vi "Get Label Text and Index.vi"(0 "Label Text and Index":string) -> (4 "Label Text and Index (Dup)":string, 8 "Text":string, 15 "Index":i32)   [LabVIEW 2016]
uses:
  <vilib>/regexp/Match Regular Expression.xnode
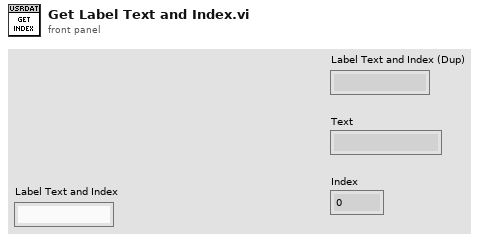
[diagram p1: front panel]
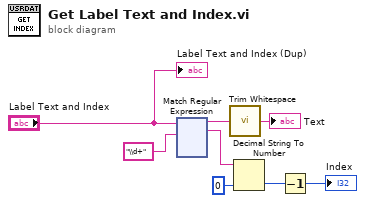
[diagram p0: block diagram]
diagram:
  n1 = xnode "Match Regular Expression"("input string"="Label Text and Index", "regular expression"="\\d+") -> ("before match"=w8:string, "whole match"=w3:string)  [unwired: 4 in, 3 out]
  n2 = call <vilib>:"Trim Whitespace.vi"("string"=w8) -> ("trimmed string"=→"Text":string)  [unwired: 1 in]
  n3 = Decimal String To Number(string=w3, default (0L)=0 ("default (0 I32)")) -> (number=w5:i32)  [unwired: 1 in, 1 out]
  n4 = Decrement(x=w5) -> (x-1=→"Index":i32)
  "Label Text and Index (Dup)" <- "Label Text and Index"
